vi "FGV_Variable_EventStart.vi"(8 "error in (no error)":errorcluster caption="entrée d'erreur (pas d'erreur)", 9 "Variable":T1="$Batch$", 10 "Data In":variant, 11 "Function":T2(ring)) -> (0 "error out":errorcluster caption="sortie d'erreur", 2 "Data Out":variant, 3 "Variables":cluster{"Name":string, "Data":variant}[](array[cluster]))   [LabVIEW 2020, in "Library Core.lvlib" / "Actor_EventStart.lvlib" / "Actor_EventStart.lvclass"]
uses:
  Actors/Actor_EventStart/Actor_EventStart/Actor_EventStart.lvclass
  Commun VI/TypeDef/Variable Printable.ctl
  Commun VI/TypeDef/Liste Error.ctl
  Commun VI/Library Commun.lvlib
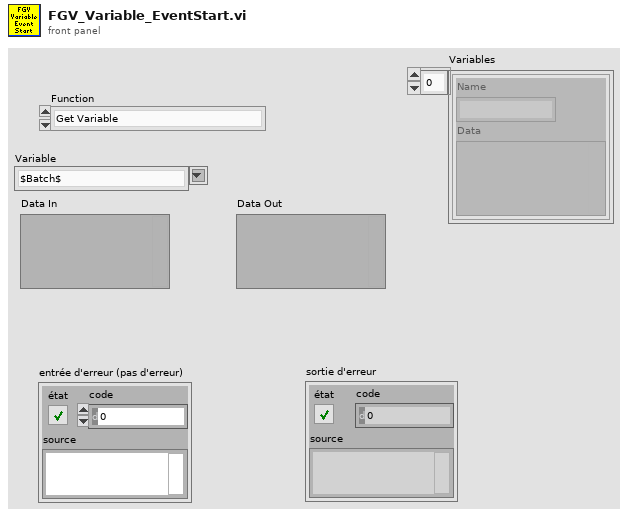
[diagram p1: front panel]
types:
  T1 = typedef "Variable Printable.ctl" = string
  T2 = enum16{"Get Variable", "Get All Variables", "Set Variable", "Delete Variable", "Delete All Variable"}
  T3 = typedef "Library Commun.lvlib/Liste Error.ctl" = enum16{"Firebase Driver - Get Document", "Firebase Driver - Get Document With Where", "Firebase Driver - Delete Document", "Firebase Driver - Set Document", "Firebase Driver - Update Document", "Firebase Altyor - Search Document Bench", "Firebase Altyor - Class Not in Firebase", "Spectrum_Analyser - Timeout", "Relay Board - Qty Relay", "DIO - Pb Funtion", "Power_Supply - Peripherical not find", "Mutimeter - Peripherical not find", "Instrument - Function Not Used", "Instrument - Instrument name not specified", "Instrument - Allready Initialised", "Instrument - TimeOut", "Instrument - the instrument must be Initialise before", "Instrument - Frame Not received", "Instrument - Frame Nok", "Test - Initialise the File_for_Save", "Test - Timeout", "Test - Cmd Error", "FGV - Variable ", "BDD FireBase - Define Class", "SN - Class Not Define"}
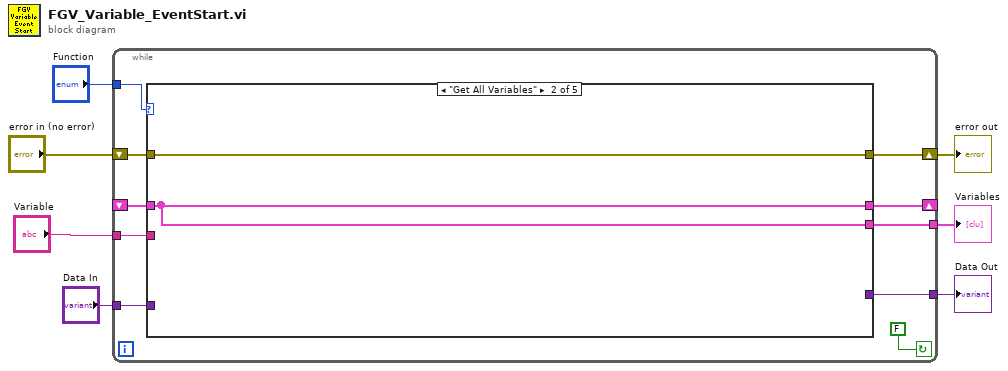
[diagram p0: block diagram]
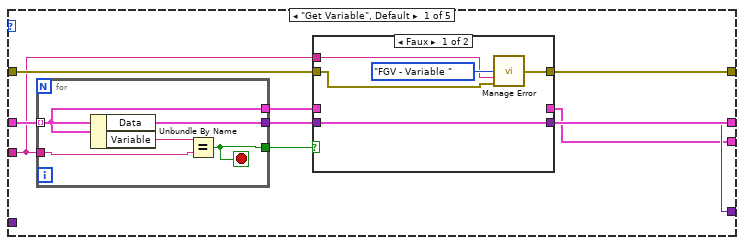
[diagram p2: hidden frame]
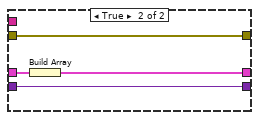
[diagram p3: hidden frame]
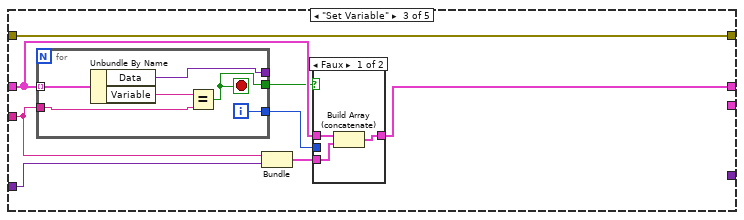
[diagram p4: hidden frame]
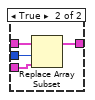
[diagram p5: hidden frame]
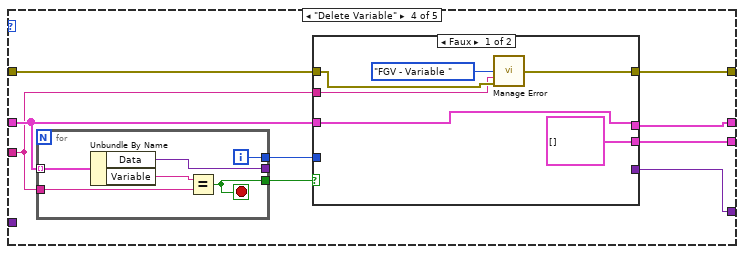
[diagram p6: hidden frame]
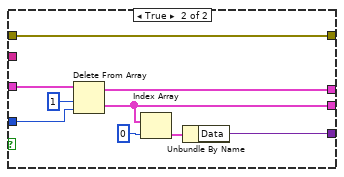
[diagram p7: hidden frame]
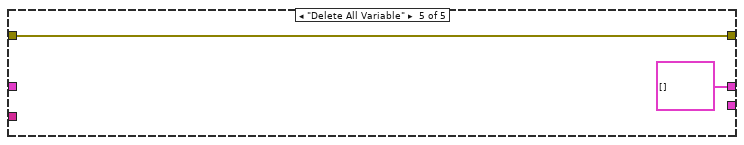
[diagram p8: hidden frame]
diagram:
  n1 = while {
    tunnel: "Function" -> [w16]
    shift-right: [w13] -> _
    shift-left: _ -> [w14]
    shift-right: [w12] -> w4
    shift-left: "error in (no error)" -> [w11]
    tunnel: [w15] -> w5
    tunnel: "Variable" -> [w10]
    tunnel: [w9] -> w2
    tunnel: "Data In" -> [w8]
    stop <- FALSE continue-if-true
    n2 = case shown="\"Get All Variables\"" w16 {
      tunnel: [w20 w41 _ w67 _] -> w15
      tunnel: w14 -> [w26 w41 w46 w70 _]
      tunnel: [w26 w41 w47 w71 cluster{"Name":string, "Data":variant}[] [] ("Variables")] -> w13
      tunnel: [w23 w40 w49 w64 w93] -> w12
      tunnel: w11 -> [w24 w40 w49 w65 w93]
      tunnel: w10 -> [w18 _ w45 w63 _]
      tunnel: [w21 _ _ w66 _] -> w9
      tunnel: w8 -> [_ _ w48 _ _]
      frame "Get Variable", Default {
        n3 = for {
          tunnel: w26 -> [w35] mode=indexing
          tunnel: w18 -> [w38]
          tunnel: [w37] -> w22
          tunnel: [w36] -> w25
          tunnel: [w35] -> w19
          stop <- w36 stop-if-true
          n4 = Unbundle By Name(w35) -> ("Data"=w37:variant, "Variable"=w39:T1)
          n5 = Equal?(x=w39, y=w38) -> (x = y?=w36:bool)
        }
        n6 = case shown="Faux" w25 {
          tunnel: w24 -> [w28 w34]
          tunnel: [w30 w34] -> w23
          tunnel: [_ w33] -> w21
          tunnel: w22 -> [_ w33]
          tunnel: [_ w31] -> w20
          tunnel: w19 -> [_ w32]
          tunnel: w18 -> [w27 _]
          frame False {
            n7 = call "Manage Error.vi"("Code Erreur"=Liste_Error."FGV - Variable ", "Text"=w27, "error in (no error)"=w28) -> ("error out"=w30:errorcluster)  [unwired: 12 in]
          }
          frame True {
            n8 = Build Array(w32) -> (w31:cluster{"Variable":T1, "Data":variant}[])
          }
        }
      }
      frame "Get All Variables" {
      }
      frame "Set Variable" {
        n9 = for {
          tunnel: w46 -> [w62] mode=indexing
          tunnel: w45 -> [w60]
          tunnel: [w59] -> _
          tunnel: [w58] -> w44
          tunnel: [w57] -> w42
          i -> [w57]
          stop <- w58 stop-if-true
          n10 = Unbundle By Name(w62) -> ("Data"=w59:variant, "Variable"=w61:T1)
          n11 = Equal?(x=w61, y=w60) -> (x = y?=w58:bool)
        }
        n12 = Bundle("Variable"=w45, "Data In"=w48) -> (w43:cluster{"Variable":T1, "Data In":variant})  [unwired: 1 in]
        n13 = case shown="Faux" w44 {
          tunnel: [w52 w53] -> w47
          tunnel: w46 -> [w51 w56]
          tunnel: w43 -> [w50 w54]
          tunnel: w42 -> [_ w55]
          frame False {
            n14 = Build Array (concatenate)(w51, w50) -> (w52:cluster{"Variable":T1, "Data In":variant}[])
          }
          frame True {
            n15 = Replace Array Subset(array=w56, new element=w54, index=w55) -> (w53:cluster{"Variable":T1, "Data":variant}[])
          }
        }
      }
      frame "Delete Variable" {
        n16 = for {
          tunnel: w70 -> [w92] mode=indexing
          tunnel: w63 -> [w90]
          tunnel: [w89] -> _
          tunnel: [w88] -> w69
          tunnel: [w87] -> w68
          i -> [w87]
          stop <- w88 stop-if-true
          n17 = Unbundle By Name(w92) -> ("Data"=w89:variant, "Variable"=w91:T1)
          n18 = Equal?(x=w91, y=w90) -> (x = y?=w88:bool)
        }
        n19 = case shown="Faux" w69 {
          tunnel: [w77 w85] -> w71
          tunnel: w70 -> [w77 w86]
          tunnel: w68 -> [_ w80]
          tunnel: [cluster{"Name":string, "Data":variant}[] [] ("Variables") w84] -> w67
          tunnel: [_ w81] -> w66
          tunnel: w65 -> [w74 w78]
          tunnel: [w73 w78] -> w64
          tunnel: w63 -> [w72 _]
          frame False {
            n20 = call "Manage Error.vi"("Code Erreur"=Liste_Error."FGV - Variable ", "Text"=w72, "error in (no error)"=w74) -> ("error out"=w73:errorcluster)  [unwired: 12 in]
          }
          frame True {
            n21 = Delete From Array(array=w86, length=1 ("longueur"), index=w80) -> (deleted portion=w84:cluster{"Variable":T1, "Data":variant}[], array with subset deleted=w85:cluster{"Variable":T1, "Data":variant}[])
            n22 = Index Array(array=w84, index=0 ("indice")) -> (element=w82:cluster{"Variable":T1, "Data":variant})
            n23 = Unbundle By Name(w82) -> ("Data"=w81:variant)
          }
        }
      }
      frame "Delete All Variable" {
      }
    }
  }
  "Variables" <- w5
  "Data Out" <- w2
  "error out" <- w4
